vi "BuildFrame.vi"(10 "Data":u16[](array[numeric]) format="%x", 11 "Header":T2={"Protocol Version (8)"=3, "Command (8)"=0, "SubCommand (8)"=0, "Status (8)"=0, "Length (32)"=0, "Register Address (32)"=0, "HeaderData2 (8)"=0, "Flags (16)"=1, "HeaderData3 (8)"=0} {"Status (8)" format="%x"; "HeaderData3 (8)" format="%x"; "HeaderData2 (8)" format="%x"; "Register Address (32)" format="%4x"; "Length (32)" format="%x"; "Flags (16)" format="%x"; "SubCommand (8)" format="%x"; "Command (8)" format="%x"; "Protocol Version (8)" format="%x"}) -> (3 "FrameOut":string)   [LabVIEW 2017]
uses:
  Controls/FrameHeader.ctl
panel:
  out "Frame":u16[](array[numeric])
  in  "Preamble":u16=41452 format="%x"
  out "number":u32
  out "hex integer string":T1
  out "concatenated string (web test)":string
  out "CRC":u16 format="%x"
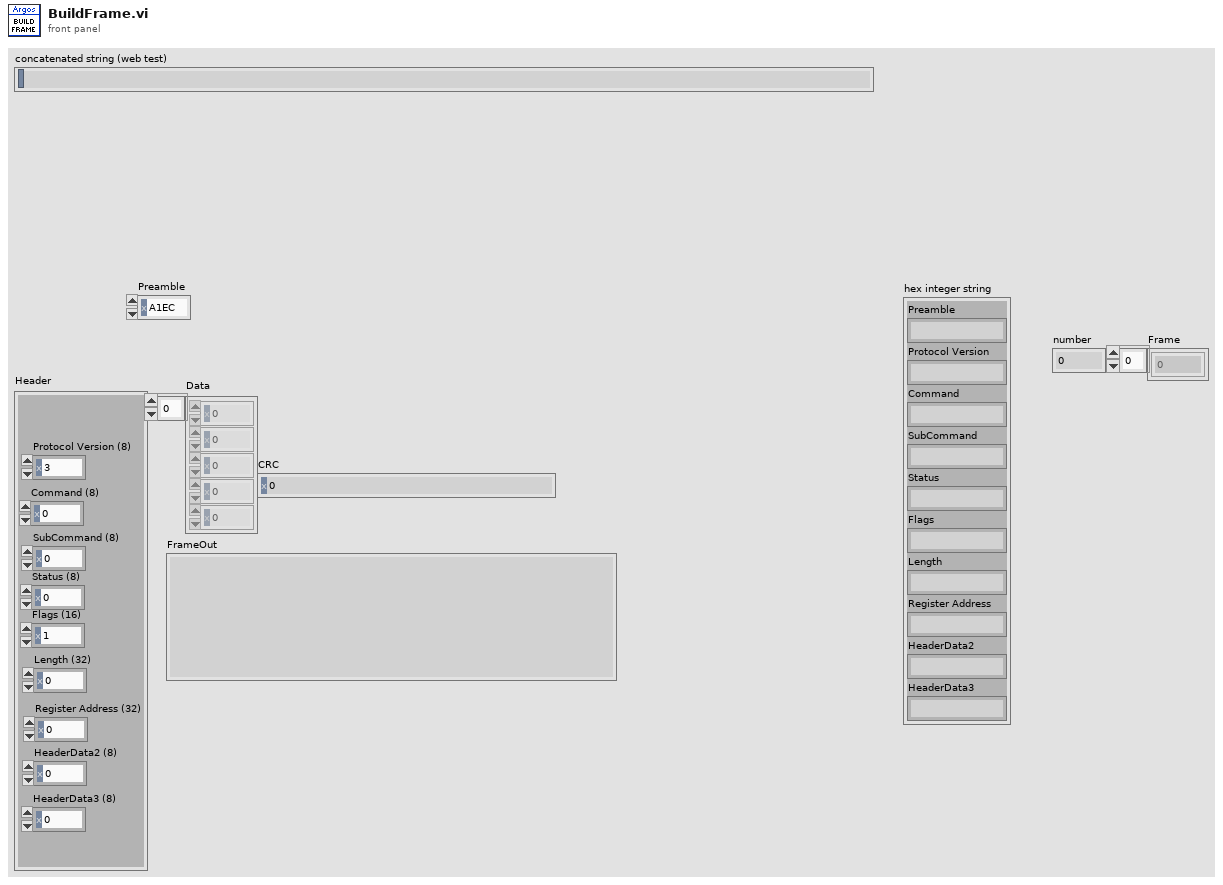
[diagram p1: front panel]
types:
  T1 = cluster{"Preamble":string, "Protocol Version":string, "Command":string, "SubCommand":string, "Status":string, "Flags":string, "Length":string, "Register Address":string, "HeaderData2":string, "HeaderData3":string}
  T2 = typedef "FrameHeader.ctl" = cluster{"Protocol Version (8)":u8, "Command (8)":u8, "SubCommand (8)":u8, "Status (8)":u8, "Length (32)":u32, "Register Address (32)":u16, "HeaderData2 (8)":u8, "Flags (16)":u16, "HeaderData3 (8)":u8}
  T3 = cluster{"Protocol Version (8)":string, "Command (8)":string, "SubCommand (8)":string, "Status (8)":string, "Length (32)":string, "Register Address (32)":string, "HeaderData2 (8)":string, "Flags (16)":string, "HeaderData3 (8)":string}
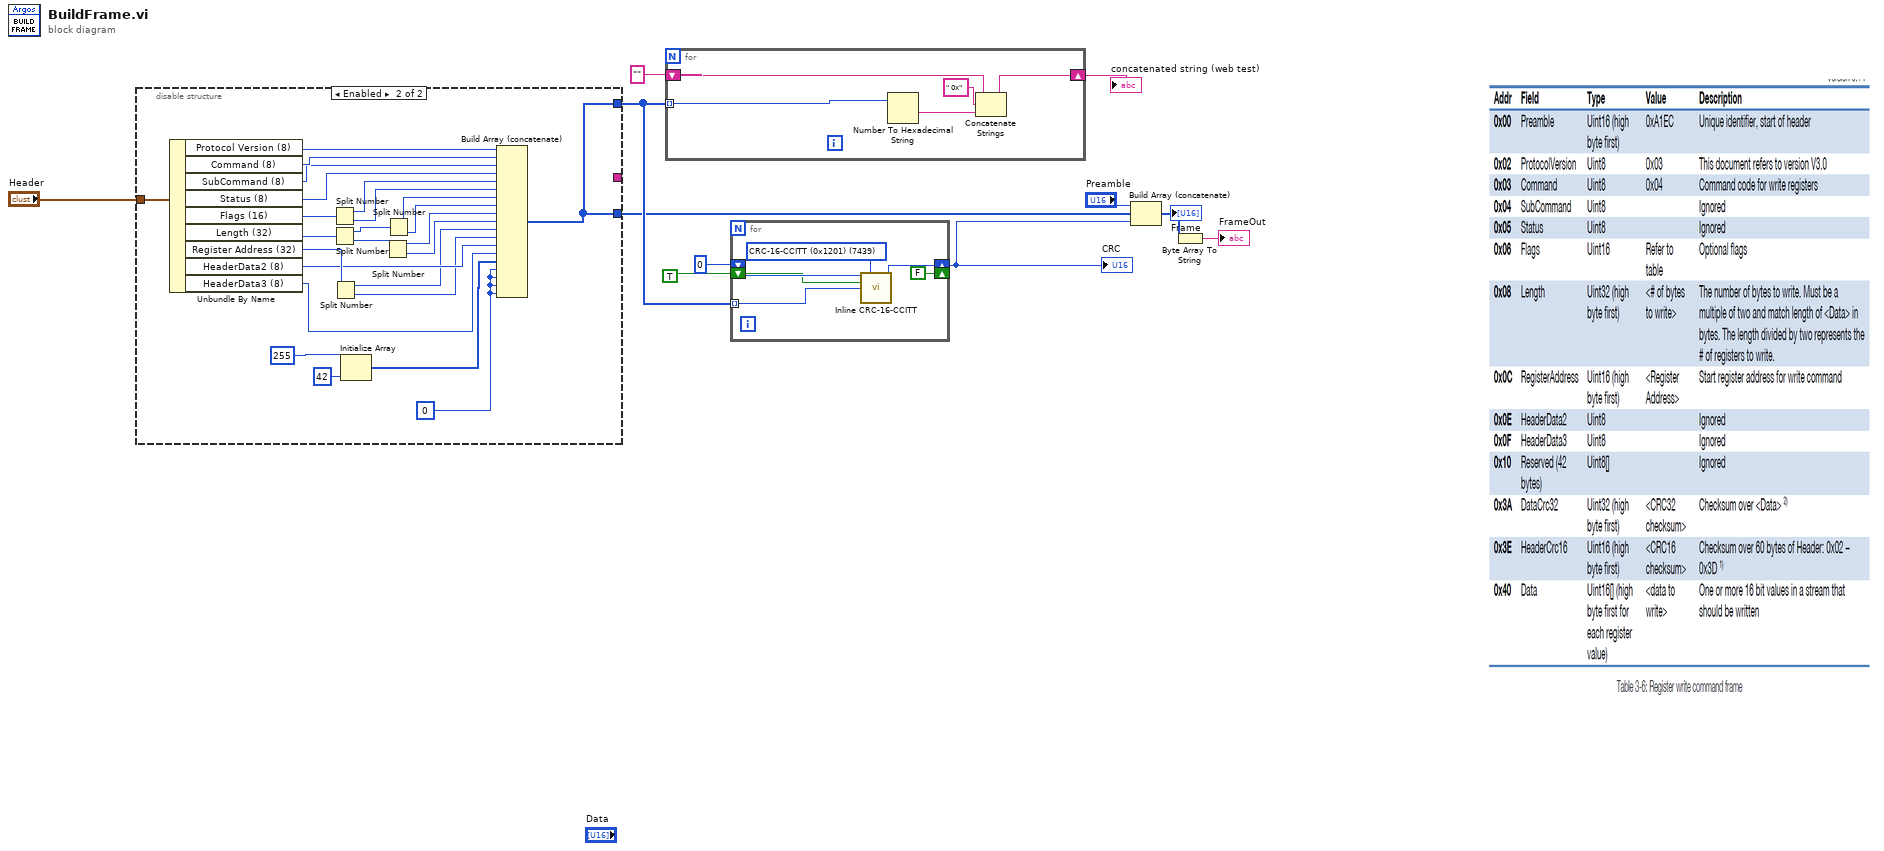
[diagram p0: block diagram]
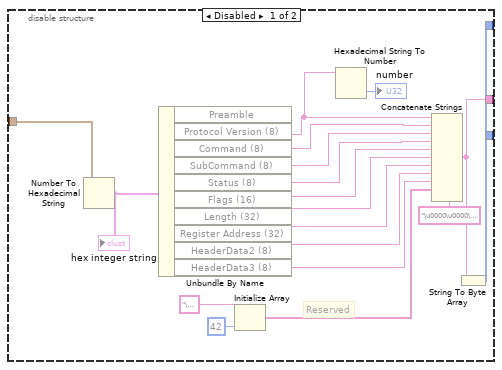
[diagram p2: hidden frame]
diagram:
  n1 = disable-structure shown="Enabled" {
    disable-tunnel: "Header" -> [w29 w54]
    disable-tunnel: [w16 _] -> _
    disable-tunnel: [w15 w30] -> w6
    disable-tunnel: [_ w30] -> w5
    frame Disabled {
      # "Reserved"
      n2 = Number To Hexadecimal String(2:w29) -> (0:w28:T3)  [unwired: 1 in]
      "hex integer string" <- w28
      n3 = Unbundle By Name(w28) -> ("Protocol Version (8)"=w13:string, "Command (8)"=w27:string, "SubCommand (8)"=w26:string, "Status (8)"=w25:string, "Flags (16)"=w24:string, "Length (32)"=w23:string, "Register Address (32)"=w22:string, "HeaderData2 (8)"=w21:string, "HeaderData3 (8)"=w20:string)  [unwired: 1 out]
      n4 = Initialize Array("\u0000", 42 ("dimension size")) -> (w17:string[])
      n5 = Hexadecimal String To Number(string=w13) -> (number=→"number":u32)  [unwired: 2 in, 1 out]
      n6 = Concatenate Strings(w13, w27, w26, w25, w24, w23, w22, w21, w20, w17, "\u0000\u0000\u0000\u0000") -> (w16:string)
      n7 = String To Byte Array(string=w16) -> (unsigned byte array=w15:u8[])
    }
    frame Enabled {
      w31 = u8 0
      n8 = Unbundle By Name(w54) -> ("Protocol Version (8)"=w53:u8, "Command (8)"=w52:u8, "SubCommand (8)"=w51:u8, "Status (8)"=w34:u8, "Flags (16)"=w50:u16, "Length (32)"=w49:u32, "Register Address (32)"=w40:u16, "HeaderData2 (8)"=w39:u8, "HeaderData3 (8)"=w38:u8)
      n9 = Split Number(x=w50) -> (hi(x)=w48:u8, lo(x)=w47:u8)
      n10 = Split Number(x=w49) -> (hi(x)=w46:u16, lo(x)=w45:u16)
      n11 = Split Number(x=w40) -> (hi(x)=w33:u8, lo(x)=w32:u8)
      n12 = Initialize Array(u8 255, 42 ("dimension size")) -> (w35:u8[])
      n13 = Split Number(x=w45) -> (hi(x)=w42:u8, lo(x)=w41:u8)
      n14 = Split Number(x=w46) -> (hi(x)=w44:u8, lo(x)=w43:u8)
      n15 = Build Array (concatenate)(w53, w52, w51, w34, w48, w47, w44, w43, w42, w41, w33, w32, w39, w38, w35, w31, w31, w31, w31) -> (w30:u8[])
    }
  }
  n16 = for {
    tunnel: w6 -> [w59] mode=indexing
    shift-right: [w56] -> w7
    shift-left: "" -> [w55]
    n17 = Number To Hexadecimal String(2:w59) -> (0:w58:string)  [unwired: 1 in]
    n18 = Concatenate Strings(w55, " 0x" ("string"), w58) -> (w56:string)
  }
  "concatenated string (web test)" <- w7
  n19 = for {
    tunnel: w6 -> [w64] mode=indexing
    shift-right: [w62] -> w3
    shift-left: u16 0 ("CRC") -> [w63]
    shift-right: [FALSE] -> _
    shift-left: TRUE -> [w61]
    w65 = u16 7439 items=["CRC-16-CCITT (0x1201)"=7439, "CRC-16-CCITT (0xFFFF)"=65535, "CRC-16-CCITT (XModem)"=0] ("CRC-CCITT Type")
    n20 = call <userlib>:"Inline CRC-16-CCITT.vi"("CRC In"=w63, "CRC-CCITT Type"=w65, "Reset"=w61, "Data"=w64) -> ("CRC"=w62:u16)  [unwired: 10 in, 1 out]
  }
  "CRC" <- w3
  n21 = Build Array (concatenate)("Preamble", w5, w3) -> (w2:u16[])
  "Frame" <- w2
  n22 = Byte Array To String(unsigned byte array=w2) -> (string=→"FrameOut":string)
